vi "ReadControlKey.vi"(9 "ConfigFile":T1, 10 "section":string, 11 "Control in":refnum<vi>) -> (3 "ConfigFile out":T1)   [LabVIEW 2015]
uses:
  <vilib>/Utility/config.llb/Config Data RefNum.ctl
  <vilib>/Utility/Data Type/Type Definitions/Data Type.ctl
  <vilib>/Utility/config.llb/Read Key (Path).vi
  <vilib>/Utility/config.llb/Read Key (String).vi
  <vilib>/Utility/config.llb/Read Key (Boolean).vi
  <vilib>/Utility/config.llb/Read Key (Double).vi
  <vilib>/Utility/config.llb/Read Key (I32).vi
  <vilib>/Utility/Data Type/NI_Data Type.lvlib
  <vilib>/Utility/config.llb/NI_LVConfig.lvlib
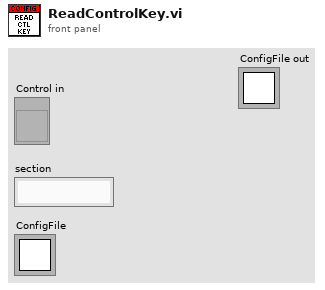
[diagram p1: front panel]
types:
  T1 = typedef "NI_LVConfig.lvlib/Config Data RefNum.ctl" = refnum<k1>
  T2 = typedef "NI_Data Type.lvlib/Data Type.ctl" = enum8{"Invalid Type", "Void", "I8", "I16", "I32", "I64", "U8", "U16", "U32", "U64", "Single Float", "Double Float", "Extended Float", "Single Complex", "Double Complex", "Extended Complex", "Enum U8", "Enum U16", "Enum U32", "Enum U64", "Single Float With Unit", "Double Float With Unit", "Extended Float With Unit", "Single Complex with Unit", "Double Complex with Unit", "Extended Complex with Unit", "Boolean", "String", "Path", "Picture", "Tag", "Array", "Cluster", "Variant", "LV Variant", "Waveform", "Timestamp", "Digital Waveform", "Digital Data", "ExpressData", "Refnum", "External Data", "VI", "Poly VI", "LabVIEW Class Instance", "Fixed Point"}
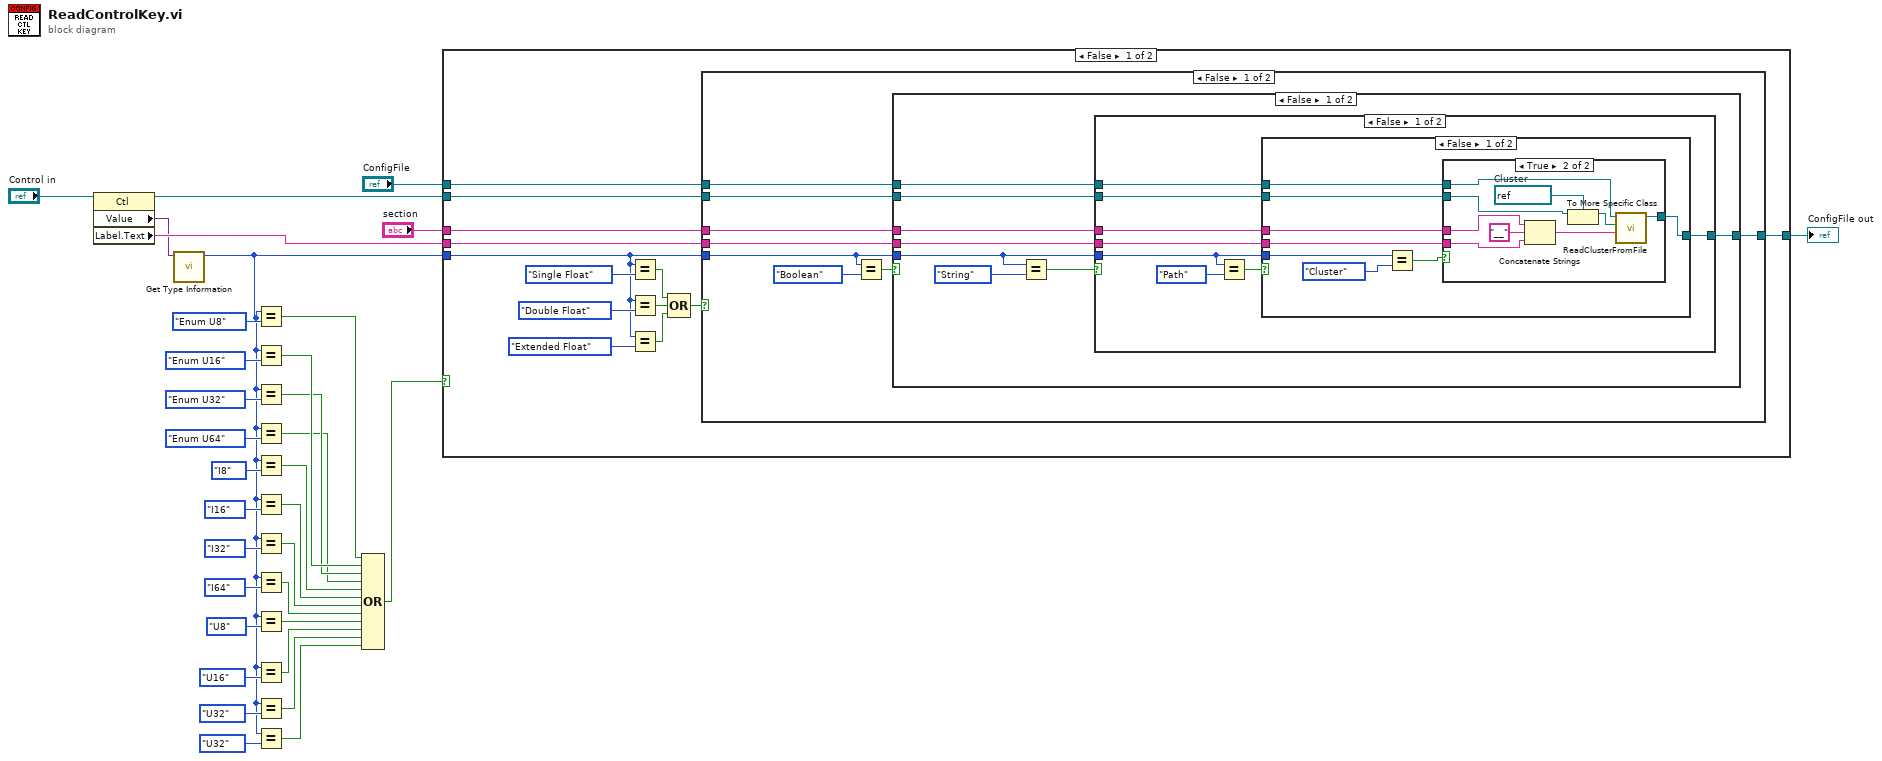
[diagram p0: block diagram]
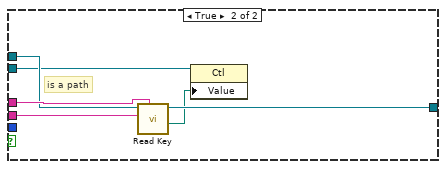
[diagram p3: hidden frame]
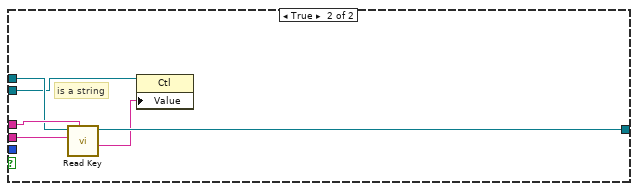
[diagram p4: hidden frame]
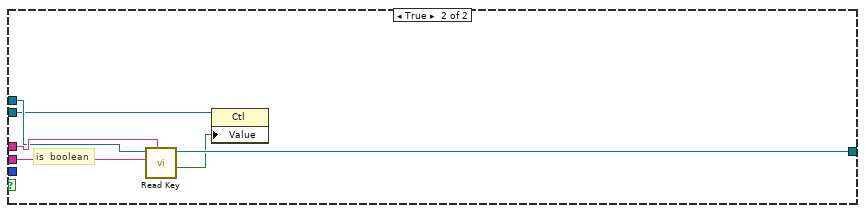
[diagram p5: hidden frame]
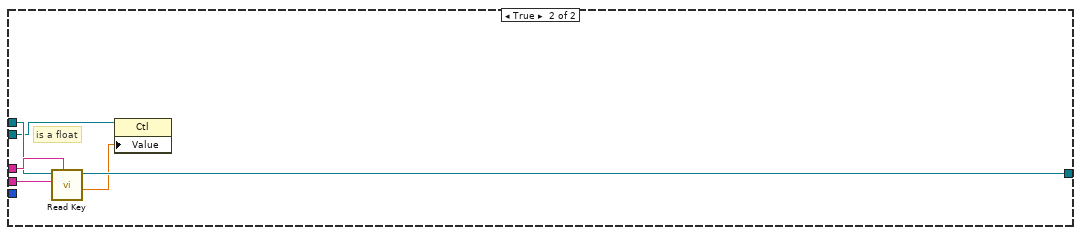
[diagram p6: hidden frame]
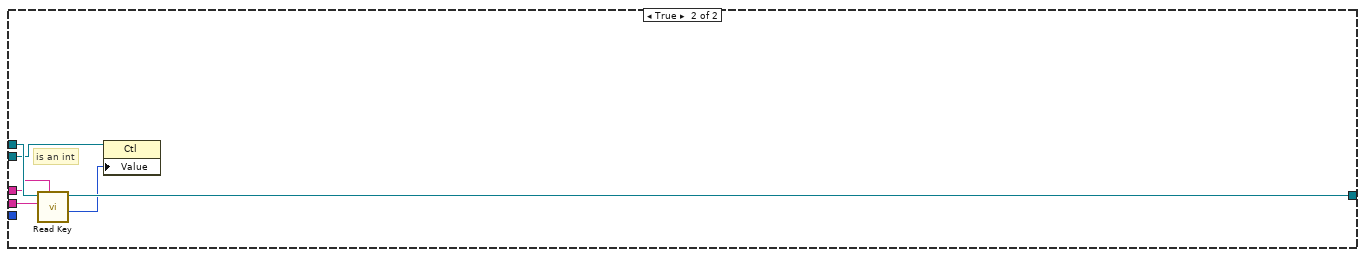
[diagram p7: hidden frame]
diagram:
  n1 = property class="Ctl"(reference="Control in") -> (reference out=w27:refnum<vi>, "Value"=w30:variant, "Label.Text"=w31:string)  [unwired: 1 in, 1 out]
  n2 = call <vilib>:"Get Type Information.vi"("Variant"=w30) -> ("Type"=w2:T2)  [unwired: 6 in, 4 out]
  n3 = Equal?(x=w2, y=Data_Type."Enum U8" ("Type")) -> (x = y?=w6:bool)
  n4 = Equal?(x=w2, y=Data_Type."Enum U16" ("Type")) -> (x = y?=w5:bool)
  n5 = Equal?(x=w2, y=Data_Type."Enum U32" ("Type")) -> (x = y?=w4:bool)
  n6 = Equal?(x=w2, y=Data_Type."Enum U64" ("Type")) -> (x = y?=w3:bool)
  n7 = Equal?(x=w2, y=Data_Type."I8" ("Type")) -> (x = y?=w19:bool)
  n8 = Equal?(x=w2, y=Data_Type."I16" ("Type")) -> (x = y?=w20:bool)
  n9 = Equal?(x=w2, y=Data_Type."I32" ("Type")) -> (x = y?=w21:bool)
  n10 = Equal?(x=w2, y=Data_Type."I64" ("Type")) -> (x = y?=w22:bool)
  n11 = Equal?(x=w2, y=Data_Type."U8" ("Type")) -> (x = y?=w23:bool)
  n12 = Equal?(x=w2, y=Data_Type."U16" ("Type")) -> (x = y?=w24:bool)
  n13 = Equal?(x=w2, y=Data_Type."U32" ("Type")) -> (x = y?=w25:bool)
  n14 = Equal?(x=w2, y=Data_Type."U32" ("Type")) -> (x = y?=w26:bool)
  n15 = Compound Arithmetic op=OR(w6, w5, w4, w3, w19, w20, w21, w22, w23, w24, w25, w26) -> (w1:bool)
  n16 = case shown="False" w1 {
    tunnel: w2 -> [w39 _]
    tunnel: w31 -> [w38 w117]
    tunnel: "ConfigFile" -> [w36 w118]
    tunnel: "section" -> [w37 w116]
    tunnel: [w35 w115] -> w28
    tunnel: w27 -> [w34 w113]
    frame False {
      n17 = Equal?(x=w39, y=Data_Type."Single Float" ("Type")) -> (x = y?=w43:bool)
      n18 = Equal?(x=w39, y=Data_Type."Double Float" ("Type")) -> (x = y?=w42:bool)
      n19 = Equal?(x=w39, y=Data_Type."Extended Float" ("Type")) -> (x = y?=w41:bool)
      n20 = Compound Arithmetic op=OR(w43, w42, w41) -> (w40:bool)
      n21 = case shown="False" w40 {
        tunnel: w39 -> [w52 _]
        tunnel: w38 -> [w51 w111]
        tunnel: w37 -> [w50 w112]
        tunnel: w36 -> [w49 w110]
        tunnel: [w48 w109] -> w35
        tunnel: w34 -> [w47 w107]
        frame False {
          n22 = Equal?(x=w52, y=Data_Type."Boolean" ("Type")) -> (x = y?=w53:bool)
          n23 = case shown="False" w53 {
            tunnel: w52 -> [w60 _]
            tunnel: w51 -> [w59 w104]
            tunnel: w50 -> [w58 w106]
            tunnel: w49 -> [w57 w105]
            tunnel: [w56 w103] -> w48
            tunnel: w47 -> [w55 w101]
            frame False {
              n24 = Equal?(x=w60, y=Data_Type."String" ("Type")) -> (x = y?=w61:bool)
              n25 = case shown="False" w61 {
                tunnel: w60 -> [w63 _]
                tunnel: w59 -> [w68 w98]
                tunnel: w58 -> [w67 w100]
                tunnel: w57 -> [w66 w99]
                tunnel: [w65 w97] -> w56
                tunnel: w55 -> [w64 w96]
                frame False {
                  n26 = Equal?(x=w63, y=Data_Type."Path" ("Type")) -> (x = y?=w69:bool)
                  n27 = case shown="False" w69 {
                    tunnel: w68 -> [w73 w92]
                    tunnel: w67 -> [w75 w94]
                    tunnel: w66 -> [w74 w93]
                    tunnel: [w71 w91] -> w65
                    tunnel: w64 -> [w72 w90]
                    tunnel: w63 -> [w77 _]
                    frame False {
                      n28 = Equal?(x=w77, y=Data_Type."Cluster" ("Type")) -> (x = y?=w76:bool)
                      n29 = case shown="True" w76 {
                        tunnel: w75 -> [_ w87]
                        tunnel: w74 -> [w79 w83]
                        tunnel: w73 -> [_ w86]
                        tunnel: w72 -> [_ w81]
                        tunnel: [w79 w84] -> w71
                        frame False {
                        }
                        frame True {
                          w82 = refnum<vi> refnum  # Cluster
                          n30 = Concatenate Strings(w87, "__" ("string"), w86) -> (w85:string)
                          n31 = To More Specific Class(target class=w82, reference=w81) -> (specific class reference=w80:refnum<vi>)  [unwired: 1 in, 1 out]
                          n32 = call "ReadClusterFromFile.vi"("Name"=w85, "Cluster in"=w80, "ConfigIn"=w83) -> ("ConfigOut"=w84:T1)  [unwired: 8 in]
                        }
                      }
                    }
                    frame True {
                      # "is a path"
                      n33 = call-poly <vilib>:"Read Key.vi"("section"=w94, "key"=w92, "refnum"=w93) -> ("value"=w89:path, "refnum out"=w91:T1)  [unwired: 5 in, 2 out]
                      n34 = property class="Ctl"(reference=w90, "Value"=w89) -> ()  [unwired: 1 in, 2 out]
                    }
                  }
                }
                frame True {
                  # "is a string"
                  n35 = call-poly <vilib>:"Read Key.vi"("section"=w100, "key"=w98, "refnum"=w99) -> ("value"=w95:string, "refnum out"=w97:T1)  [unwired: 5 in, 2 out]
                  n36 = property class="Ctl"(reference=w96, "Value"=w95) -> ()  [unwired: 1 in, 2 out]
                }
              }
            }
            frame True {
              # "is  boolean"
              n37 = call-poly <vilib>:"Read Key.vi"("section"=w106, "key"=w104, "refnum"=w105) -> ("value"=w102:bool, "refnum out"=w103:T1)  [unwired: 5 in, 2 out]
              n38 = property class="Ctl"(reference=w101, "Value"=w102) -> ()  [unwired: 1 in, 2 out]
            }
          }
        }
        frame True {
          # "is a float"
          n39 = call-poly <vilib>:"Read Key.vi"("section"=w112, "key"=w111, "refnum"=w110) -> ("value"=w108:dbl, "refnum out"=w109:T1)  [unwired: 5 in, 2 out]
          n40 = property class="Ctl"(reference=w107, "Value"=w108) -> ()  [unwired: 1 in, 2 out]
        }
      }
    }
    frame True {
      # "is an int"
      n41 = call-poly <vilib>:"Read Key.vi"("section"=w116, "key"=w117, "refnum"=w118) -> ("value"=w114:i32, "refnum out"=w115:T1)  [unwired: 5 in, 2 out]
      n42 = property class="Ctl"(reference=w113, "Value"=w114) -> ()  [unwired: 1 in, 2 out]
    }
  }
  "ConfigFile out" <- w28
